vi "Write to Excel Worksheet.vi"(7 "Worksheet":string="Raw Data", 8 "error in (no error)":errorcluster, 9 "File Out Path":path, 10 "Table In":string[][](array[string]), 11 "Template Path":path=path "C:/ER2006/Excel Data/ER Template.xls") -> (0 "error out":errorcluster)   [LabVIEW 2013]
doc: "Write data to reports worksheet."
uses:
  <vilib>/Utility/NIReport.llb/NI_report.lvclass
  <vilib>/Utility/NIReport.llb/Append Text Table to Report (wrap).vi
  <vilib>/Utility/NIReport.llb/Excel/NI_Excel.lvclass
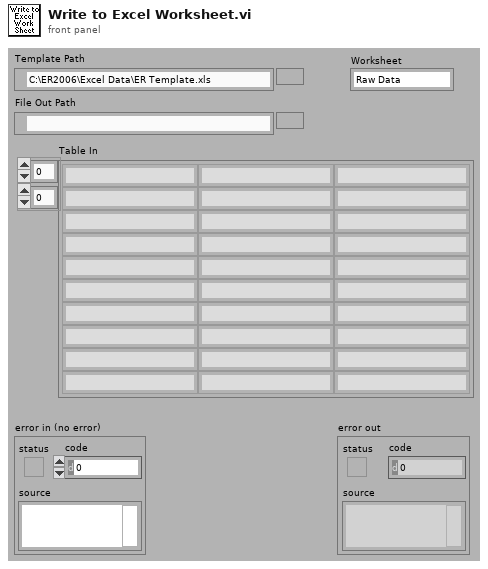
[diagram p1: front panel]
types:
  T1 = enum16{"maximized", "minimized", "normal", "no change"}
  T2 = enum16{"Standard Report", "HTML", "Word", "Excel"}
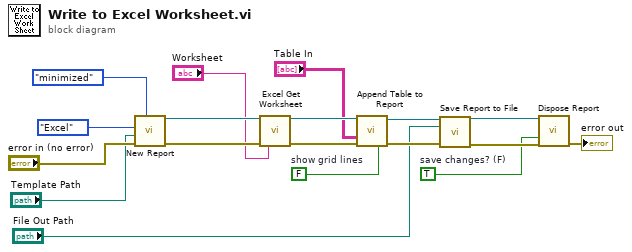
[diagram p0: block diagram]
diagram:
  w7 = TRUE  # save changes? (F)
  w8 = FALSE  # show grid lines
  n1 = call <vilib>:"New Report.vi"("window state (normal)"=T1."minimized", "report type"=T2."Excel", "template (empty)"="Template Path", "error in (no error)"="error in (no error)") -> ("report out"=w5:refnum<class "NI_report.lvclass">, "error out"=w16:errorcluster)  [unwired: 10 in]
  n2 = call <vilib>:"Excel Get Worksheet.vi"("report in"=w5, "error in (no error)"=w16, "name (\"\")"="Worksheet") -> ("report out"=w14:refnum<class "NI_report.lvclass">, "error out"=w15:errorcluster)  [unwired: 11 in]
  n3 = call-poly <vilib>:"Append Table to Report.vi"("report in"=w14, "text data"="Table In", "error in (no error)"=w15, "show grid lines (YES)"=w8) -> ("report out"=w12:refnum<class "NI_report.lvclass">, "error out"=w13:errorcluster)  [unwired: 8 in, 2 out]
  n4 = call-dynamic "Save Report to File.vi"("report in"=w12, "report file path"="File Out Path", "error in (no error)"=w13) -> ("report out"=w10:refnum<class "NI_report.lvclass">, "error out"=w11:errorcluster)  [unwired: 11 in]
  n5 = call-dynamic "Dispose Report.vi"("report in"=w10, "save changes? (F)"=w7, "error in (no error)"=w11) -> ("error out"=→"error out":errorcluster)  [unwired: 12 in]
